vi "Generation Engine.vi"(6 "User-defined Start Trigger - AO":bool, 8 "dsp config":T1, 9 "config in":T4, 10 "linked start trigger from ai":bool, 11 "fifo from host":refnum<k21>) -> (2 "state out":T3, 3 "data to IO node":cluster{"ao1":fxp<+/-,12,1>[]}[](array[cluster]))   [LabVIEW 2018, in "GettingStarted_5785_FPGA.lvlib"]
uses:
  GettingStarted_5785_FPGA.lvlib
  Generation Engine Cfg.ctl
  <instrlib>/_niInstr/Streaming/v1/Common/Stream State.ctl
  <instrlib>/FlexRIO/API/FPGA/v1/IO/NI5785/AO DSP Cfg.ctl
  <instrlib>/FlexRIO/API/FPGA/v1/Types/Start Trigger IO Resources.ctl
  <vilib>/rvi/DataTransferAndStorage/Container/Common/niFpgaContainerExecOnDevCompGetState.vi
  <vilib>/rvi/Emulation/niFpgaEmulationIsFPGAContextNoSignature.vi
  <vilib>/rvi/Emulation/niFpgaSctlEmulationGetInTimedLoop.vi
  <vilib>/rvi/errors/niFpgaSetErrorForExecOnDevCompSimple.vi
  <vilib>/rvi/eio/common/nirviEmuReportErrorAndStop.vi
  <vilib>/rvi/DataTransferAndStorage/Container/Common/niFpgaContainerGetUniqueNameForEmu.vi
  <vilib>/rvi/FIFO/Fifo_Resource/nirvififoEmulationSetSize.vi
  <vilib>/rvi/FIFO/Fifo_Resource/nirviFifoEmulationQueueMgr.vi
  <instcachedir>/0/nirviFifoEmulationQueueMgr_E5CAEC123FF24DC58D834DCA3CDAA9B5.lvgen/nirviFifoEmulationQueueMgr_E5CAEC123FF24DC58D834DCA3CDAA9B5_015.vi
  <vilib>/rvi/FIFO/Fifo_Resource/nirvififoEmulationDetermineInputValidOut.vi
  <vilib>/rvi/FIFO/Fifo_Resource/nirvififoEmulationCreateLock.vi
  <vilib>/rvi/Emulation/niFpgaProcessEmulError.vi
  <vilib>/rvi/FIFO/Fifo_Resource/nirvififoEmulationObtainLock.vi
  <vilib>/rvi/FIFO/Fifo_Resource/nirvififoEmulationReleaseLock.vi
  <vilib>/rvi/occurrence/nirviWaitOnOccurrenceBase.vi
  <vilib>/rvi/errors/nirviReportUnexpectedCaseInternalError.vi
  <vilib>/rvi/errors/nirviReportUnexpectedCaseInternalError (U32).vi
  <vilib>/Utility/error.llb/Clear Errors.vi
  <vilib>/rvi/interface/RandomDataEmulation/niFpgaRandomDataHandleErrors.vi
  2cd06dc4-3ec7-4f72-b4bb-721458c6efc6.vi
  <vilib>/rvi/DataTransferAndStorage/Container/XNode/niFpgaContainer.xnode
  <vilib>/rvi/FIFO/Fifo_Resource/niFpgaFifoEmulationRefIn.vi
  <instrlib>/_niInstr/Streaming/v1/FPGA/niInstr Streaming v1 FPGA.lvlib
  <instrlib>/FlexRIO/API/FPGA/v1/FlexRIO API FPGA v1.lvlib
  <instrlib>/FlexRIO/API/FPGA/v1/IO/NI5785/FlexRIO 5785 FPGA v1.lvlib
  <instrlib>/_niInstr/Streaming/v1/Common/niInstr Streaming v1 Common.lvlib
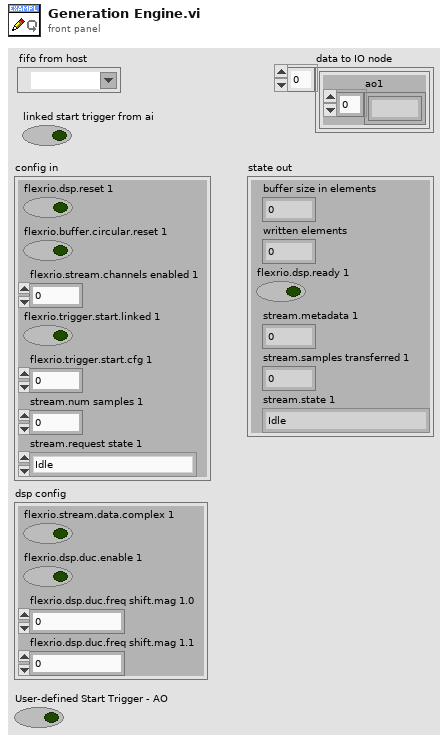
[diagram p1: front panel]
types:
  T1 = typedef "FlexRIO 5785 FPGA v1.lvlib/AO DSP Cfg.ctl" = cluster{"flexrio.stream.data.complex 1":bool, "flexrio.dsp.duc.enable 1":bool, "flexrio.dsp.duc.freq shift.mag 1.0":fxp<+/-,48,0>, "flexrio.dsp.duc.freq shift.mag 1.1":fxp<+/-,48,0>}
  T2 = typedef "niInstr Streaming v1 Common.lvlib/Stream State.ctl" = enum8{"Idle", "Finite Transfer", "Continuous", "Done", "Error", "Not Ready", "Cancel"}
  T3 = cluster{"buffer size in elements":u64, "written elements":u64, "flexrio.dsp.ready 1":bool, "stream.metadata 1":u64, "stream.samples transferred 1":u64, "stream.state 1":T2}
  T4 = typedef "GettingStarted_5785_FPGA.lvlib/Generation Engine Cfg.ctl" = cluster{"flexrio.dsp.reset 1":bool, "flexrio.buffer.circular.reset 1":bool, "flexrio.stream.channels enabled 1":u64, "flexrio.trigger.start.linked 1":bool, "flexrio.trigger.start.cfg 1":u16, "stream.num samples 1":u64, "stream.request state 1":T2}
  T5 = typedef "FlexRIO API FPGA v1.lvlib/Start Trigger IO Resources.ctl" = cluster{"start trigger":refnum<k21>, "started event":refnum<k21>, "start trigger for export":refnum<k21>, "start trigger for tclk":refnum<k21>}
  T6 = typedef "FlexRIO API FPGA v1.lvlib/Start Trigger Control.ctl" = cluster{"arm start":bool, "done":bool}
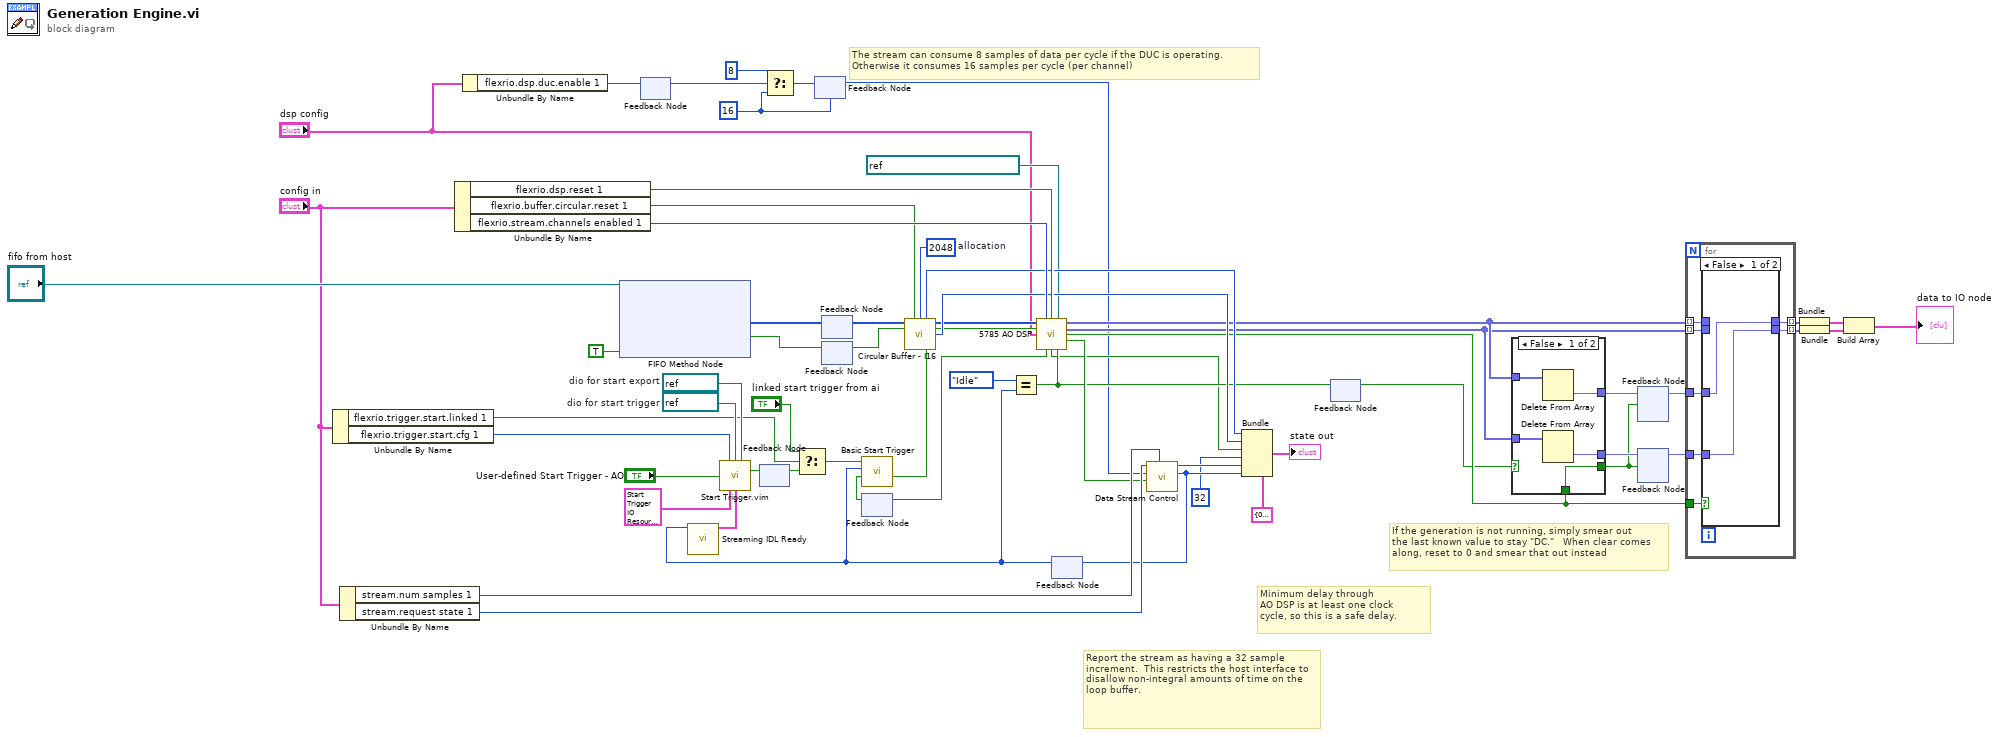
[diagram p0: block diagram]
diagram:
  w6 = u16 16 ("element count")
  w39 = refnum<k21> "DIO 2"  # dio for start trigger
  w40 = refnum<k21> "DIO 3"  # dio for start export
  w32 = 2048  # allocation
  # "The stream can consume 8 samples of data per cycle if the DUC is operating.  Otherwise it consumes 16 samples per cycle (per channel)"
  # "Report the stream as having a 32 sample increment.  This restricts the host interface to disallow non-integral amounts of time on the loop buffer."
  # "Minimum delay through\nAO DSP is at least one clock\ncycle, so this is a safe delay."
  # "If the generation is not running, simply smear out\nthe last known value to stay \"DC.\"   When clear comes along, reset to 0 and smear that out instead"
  n1 = Unbundle By Name("config in") -> ("flexrio.trigger.start.linked 1"=w26:bool, "flexrio.trigger.start.cfg 1"=w25:u16)
  n2 = Unbundle By Name("config in") -> ("stream.num samples 1"=w62:u64, "stream.request state 1"=w63:T2)
  n3 = Unbundle By Name("config in") -> ("flexrio.dsp.reset 1"=w58:bool, "flexrio.buffer.circular.reset 1"=w59:bool, "flexrio.stream.channels enabled 1"=w60:u64)
  n4 = Unbundle By Name("dsp config") -> ("flexrio.dsp.duc.enable 1"=w4:bool)
  n5 = xnode ("FIFO Method Node")("Ready for Output"=TRUE, "FIFO In"="fifo from host") -> ("Element"=w31:i16[], "Output Valid"=w29:bool)  [unwired: 1 out]
  n6 = feedback-in #1(w4) -> ()
  n7 = feedback #1() -> (w3:bool)  [unwired: 1 in]
  n8 = feedback #2() -> (w52:bool)  [unwired: 1 in]
  n9 = Select(t=u16 8 ("element count"), s=w3, f=w6) -> (s? t:f=w5:u16)
  n10 = Select(t="linked start trigger from ai", s=w26, f=w52) -> (s? t:f=w35:bool)
  n11 = feedback-in #3(w5) -> ()
  n12 = feedback #3(w6) -> (w1:u16)
  n13 = feedback #4() -> (w50:i16[])  [unwired: 1 in]
  n14 = feedback-in #4(w31) -> ()
  n15 = feedback #5() -> (w51:bool)  [unwired: 1 in]
  n16 = feedback-in #5(w29) -> ()
  n17 = feedback #6() -> (w47:bool)  [unwired: 1 in]
  n18 = feedback #7() -> (w45:T2)  [unwired: 1 in]
  n19 = call <instrlib>:"Streaming IDL Ready.vi"("stream.state"=w45) -> ("start trigger control"=w37:T6)  [unwired: 10 in]
  n20 = call "Start Trigger.vim"("flexrio.trigger.start.cfg 0"=w25, "dio start"=w39, "dio for start export"=w40, "user-defined start trigger"="User-defined Start Trigger - AO", "trigger io resources"=T5 {"start trigger"="Routing\\StartTrigger1", "started event"="Routing\\StartedEvent1", "start trigger for export"="Routing\\StartTriggerForExport1", "start trigger for tclk"="Routing\\StartTriggerForTClk1"}, "start trigger control"=w37) -> ("conditioned start trigger"=w38:bool)  [unwired: 7 in, 2 out]
  n21 = feedback-in #2(w38) -> ()
  n22 = call <instrlib>:"Basic Start Trigger.vi"("data valid?"=w47, "stream.state"=w45, "start trigger"=w35) -> ("data valid"=w33:bool)  [unwired: 8 in]
  n23 = call <instrlib>:"Circular Buffer - I16.vi"("write data"=w50, "reset"=w59, "allocation (clock cycles)"=w32, "write data valid"=w51, "ready for output"=w33) -> ("buffer size in elements"=w54:u64, "read data"=w53:i16[], "read data valid"=w28:bool, "written elements"=w55:u64)  [unwired: 7 in]
  n24 = Equal?(x=Stream_State."Idle" ("stream.state"), y=w45) -> (x = y?=w13:bool)
  n25 = call <instrlib>:"5785 AO DSP.vi"("interleaved AO data"=w53, "flexrio.stream.channels enabled 1"=w60, "flexrio.dsp.reset 1"=w58, "clock x 2"=refnum<k21> "IO Socket\\Data Clock 2x", "data valid"=w28, "dsp config"="dsp config", "clear state"=w13) -> ("ao0"=w15:fxp<+/-,12,1>[], "ao1"=w14:fxp<+/-,12,1>[], "ao valid"=w12:bool, "data valid for engine"=w49:bool, "ready for input"=w46:bool, "flexrio.dsp.ready 1"=w8:bool)  [unwired: 3 in]
  n26 = feedback-in #6(w46) -> ()
  n27 = call <instrlib>:"Data Stream Control.vi"("stream.num samples 0"=w62, "data valid"=w49, "element count"=w1, "stream.request state 0"=w63) -> ("stream.state 0"=w42:T2, "stream.samples transferred 0"=w43:u64)  [unwired: 3 in, 3 out]
  n28 = feedback-in #7(w42) -> ()
  n29 = Bundle(cluster=T3 {"buffer size in elements"=0, "written elements"=0, "flexrio.dsp.ready 1"=FALSE, "stream.metadata 1"=0, "stream.samples transferred 1"=0, "stream.state 1"=enum."Idle"}, "buffer size in elements"=w54, "written elements"=w55, "flexrio.dsp.ready 1"=w8, "stream.metadata 1"=u64 32, "stream.samples transferred 1"=w43, "stream.state 1"=w42) -> (→"state out":T3)
  n30 = feedback-in #8(w13) -> ()
  n31 = feedback #8() -> (w10:bool)  [unwired: 1 in]
  n32 = case shown="False" w10 {
    selector: w10 -> [_ w69]
    tunnel: [w68 _] -> w22
    tunnel: [w67 _] -> w21
    tunnel: w14 -> [w66 _]
    tunnel: w15 -> [w65 _]
    tunnel: [w64 w69] -> w16
    tunnel: w12 -> [w64 _]
    frame False {
      n33 = Delete From Array(array=w65) -> (deleted portion=w68:fxp<+/-,12,1>)  [unwired: 2 in, 1 out]
      n34 = Delete From Array(array=w66) -> (deleted portion=w67:fxp<+/-,12,1>)  [unwired: 2 in, 1 out]
    }
    frame True {
    }
  }
  n35 = feedback #9() -> (w18:fxp<+/-,12,1>)  [unwired: 1 in]
  n36 = feedback-in #9(w22, w16) -> ()
  n37 = feedback #10() -> (w17:fxp<+/-,12,1>)  [unwired: 1 in]
  n38 = feedback-in #10(w21, w16) -> ()
  n39 = for {
    tunnel: w14 -> [w74] mode=indexing
    tunnel: w15 -> [w76] mode=indexing
    tunnel: [w75] -> w20 mode=indexing
    tunnel: [w73] -> w19 mode=indexing
    tunnel: w12 -> [w72]
    tunnel: w18 -> [w71]
    tunnel: w17 -> [w70]
    n40 = case shown="False" w72 {
      tunnel: [w78 w80] -> w75
      tunnel: w76 -> [_ w80]
      tunnel: w74 -> [_ w79]
      tunnel: [w77 w79] -> w73
      tunnel: w71 -> [w78 _]
      tunnel: w70 -> [w77 _]
      frame False {
      }
      frame True {
      }
    }
  }
  n41 = Bundle(w20) -> (w23:cluster{fxp<+/-,12,1>[]})  [unwired: 1 in]
  n42 = Bundle(w19) -> (w24:cluster{fxp<+/-,12,1>[]})  [unwired: 1 in]
  n43 = Build Array(w23, w24) -> (→"data to IO node":cluster{fxp<+/-,12,1>[]}[])
